vi "Set Shutter ALEX.vi"(8 "error in (no error)":errorcluster, 10 "ALEX":bool, 11 "Application in":refnum<class "Application.lvclass">) -> (0 "error out":errorcluster, 3 "Application out":refnum<class "Application.lvclass">)   [LabVIEW 2018, in "Application.lvlib" / "Application.lvclass"]
uses:
  Application.lvclass
  Application.lvclass/Application.ctl
  Hardware/Synchronization Device Messages/Set ALEX Msg/Set ALEX Msg.lvclass/Set ALEX Msg.ctl
  <vilib>/ActorFramework/Message Enqueuer/Message Enqueuer.lvclass/Message Enqueuer.ctl
  <vilib>/ActorFramework/Message Enqueuer/Enqueue.vi
  Hardware/Synchronization Device Messages/Set ALEX Msg/Set ALEX Msg.lvclass
  C:/Program Files/National Instruments/LabVIEW 2018/vi.lib/ActorFramework/Message/Message.lvclass
  <vilib>/ActorFramework/Message Priority Queue/Priority Enqueue.vi
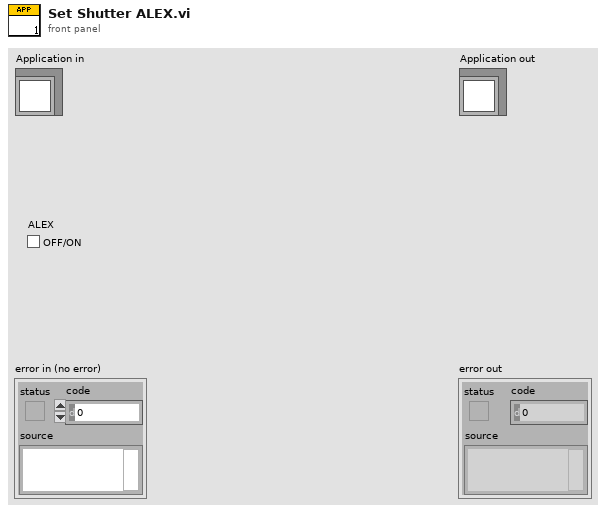
[diagram p1: front panel]
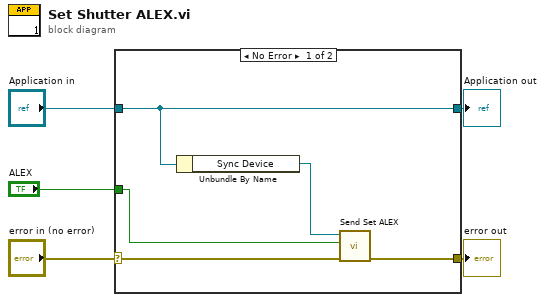
[diagram p0: block diagram]
diagram:
  n1 = case shown="No Error" "error in (no error)" {
    selector: "error in (no error)" -> [w7 w12]
    tunnel: [w6 w12] -> w4
    tunnel: [w10 w11] -> w2
    tunnel: "Application in" -> [w10 w11]
    tunnel: "ALEX" -> [w8 _]
    frame No Error {
      n2 = Unbundle By Name(w10) -> ("Sync Device"=w9:refnum<class "Message Enqueuer.lvclass">)
      n3 = call "Send Set ALEX.vi"("error in (no error)"=w7, "ALEX?"=w8, "Message Enqueuer"=w9) -> ("error out"=w6:errorcluster)  [unwired: 7 in, 1 out]
    }
    frame Error {
    }
  }
  "error out" <- w4
  "Application out" <- w2
